vi "StandardStateMachine clock2.vi"() -> ()   [LabVIEW 2014]
doc: "Use this template to build a standard state machine design pattern. Each state executes code and determines which state to transition to. Contrast this design pattern with the User Interface Event Handler pattern, in which code executes in response to user actions. Contrast this design pattern also with the Queued Message Handler pattern, in which each message handling code can queue zero or more new messages.\nNote: This template does not contain the most recent programming guidelines recommended by National Instruments. For a complete, project-based implementation of the Standard State Machine pattern, use the Create Project dialog box instead of this template."
uses:
  second v2.ctl
  minute v2.ctl
  hour v2.ctl
  StateMachineStates clock2.ctl
panel:
  in  "Stop After":i32 format="%.0f Hours"
  in  "Start":bool
  out "minute hand":T1 scale=1.0..59.0
  out "second hand":T2 scale=1.0..59.0
  out "hour hand":T3 scale=0.0..12.0
  out "x+1":i32
  out "HOUR":string
  out "MINUTE":string
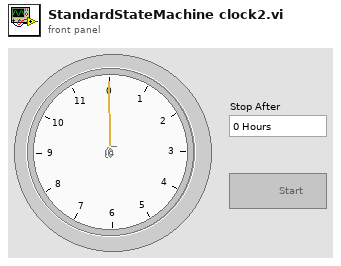
[diagram p1: front panel]
types:
  T1 = typedef "minute v2.ctl" = dbl
  T2 = typedef "second v2.ctl" = dbl
  T3 = typedef "hour v2.ctl" = dbl
  T4 = typedef "StateMachineStates clock2.ctl" = enum16{"Initialize", "normal count", "counting", "Stop"}
  T5 = enum8{"Enabled", "Disabled", "Disabled and Grayed Out"}
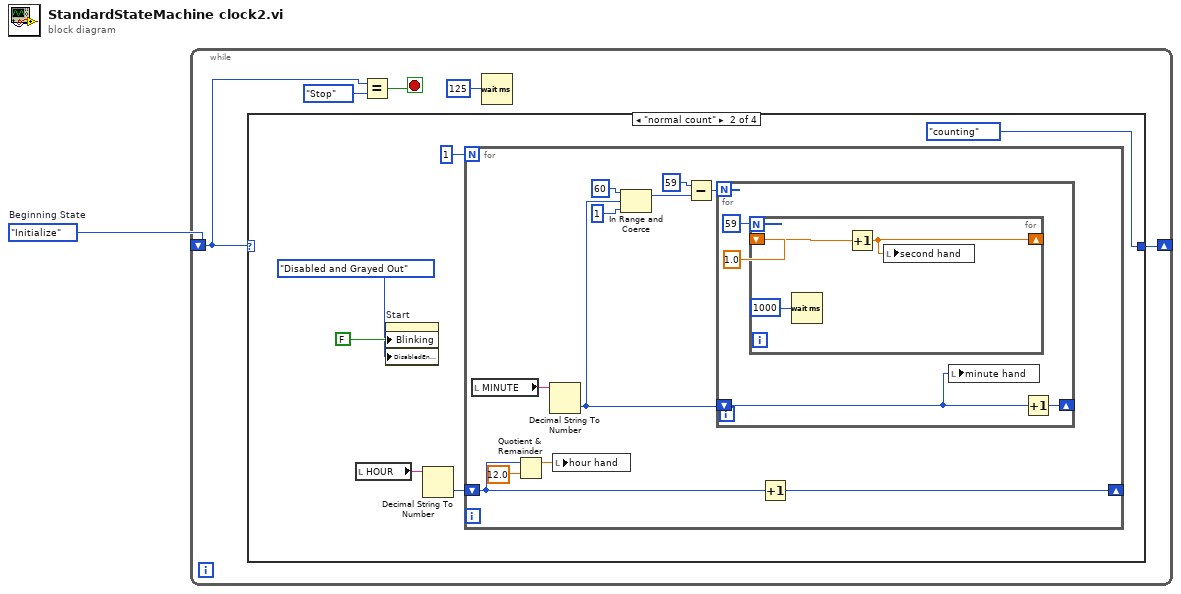
[diagram p0: block diagram]
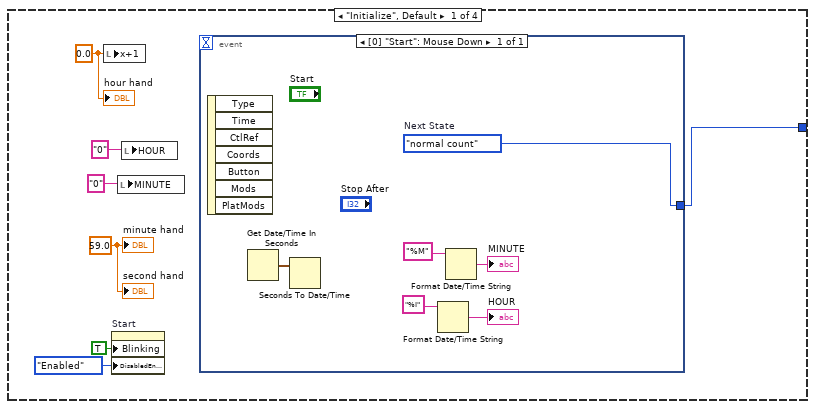
[diagram p2: hidden frame]
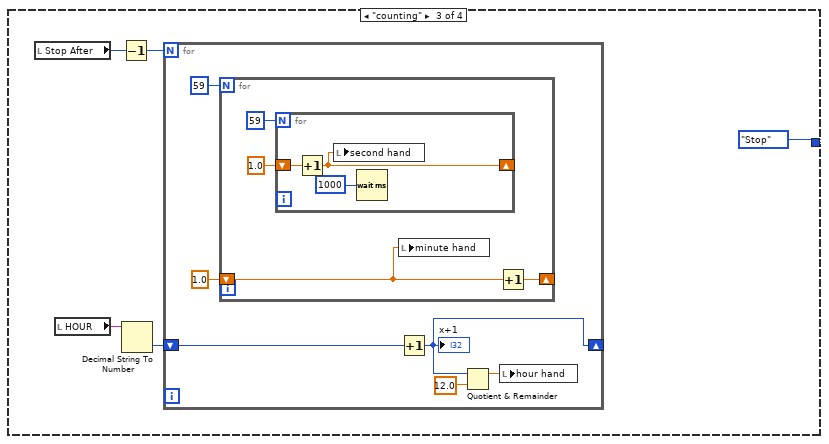
[diagram p3: hidden frame]
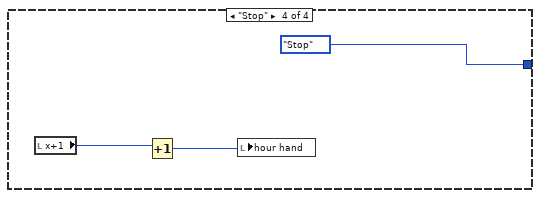
[diagram p4: hidden frame]
diagram:
  w1 = StateMachineStates_clock2."Initialize"  # Beginning State
  n1 = while {
    shift-right: [w3] -> _
    shift-left: w1 -> [w4]
    stop <- w6 stop-if-true
    n2 = case shown="\"normal count\"" w4 {
      tunnel: [w13 StateMachineStates_clock2."counting" ("Next State") StateMachineStates_clock2."Stop" ("Next State") StateMachineStates_clock2."Stop" ("Next State")] -> w3
      frame "Initialize", Default {
        w8 = T3 0.0 ("hour hand")
        w12 = T2 59.0 ("Gauge")
        n3 = local write "x+1"(w8) -> ()
        n4 = property on="Start" class="Bool (strict)"("Blinking"=TRUE ("Visible"), "DisabledEnum"=T5."Enabled" ("Disabled")) -> ()  [unwired: 2 in, 2 out]
        n5 = local write "MINUTE"("0" ("MINUTE")) -> ()
        n6 = local write "HOUR"("0" ("HOUR")) -> ()
        n7 = event shown="[0] \"Start\": Mouse Down" {
          selector: _ -> [_]
          dyn-events: _ -> [_]
          timeout: _ -> [_]
          tunnel: [w19] -> w13
          event "Start": Mouse Down {
            w19 = StateMachineStates_clock2."normal count"  # Next State
            n8 = event-data() -> ()  [unwired: 1 in, 7 out]
            n9 = Get Date/Time In Seconds() -> (seconds since 1Jan1904=w18:timestamp)
            n10 = Seconds To Date/Time(time stamp (now)=w18) -> ()  [unwired: 1 in, 1 out]
            n11 = Format Date/Time String(time format string (%c)="%I") -> (date/time string=→"HOUR":string)  [unwired: 2 in]
            n12 = Format Date/Time String(time format string (%c)="%M") -> (date/time string=→"MINUTE":string)  [unwired: 2 in]
          }
        }
        "second hand" <- w12
        "minute hand" <- w12
        "hour hand" <- w8
      }
      frame "normal count" {
        n13 = local read "HOUR"() -> (w24:string)
        n14 = property on="Start" class="Bool (strict)"("Blinking"=FALSE ("Visible"), "DisabledEnum"=T5."Disabled and Grayed Out" ("Disabled")) -> ()  [unwired: 2 in, 2 out]
        n15 = Decimal String To Number(string=w24) -> (number=w23:i32)  [unwired: 2 in, 1 out]
        n16 = for {
          N: 1 -> [_]
          shift-right: [w32] -> _
          shift-left: w23 -> [w33]
          n17 = local read "MINUTE"() -> (w34:string)
          n18 = Quotient & Remainder(x=w33, y=12.0) -> (x-y*floor(x/y)=w35:dbl)  [unwired: 1 out]
          n19 = Decimal String To Number(string=w34) -> (number=w31:i32)  [unwired: 2 in, 1 out]
          n20 = local write "hour hand"(w35) -> ()
          n21 = In Range and Coerce(upper limit=60, x=w31, lower limit=1) -> (coerced(x)=w27:i32)  [unwired: 1 out]
          n22 = Subtract(x=59 ("y"), y=w27) -> (x-y=w28:i32)
          n23 = for {
            N: w28 -> [_]
            shift-right: [w39] -> _
            shift-left: w31 -> [w40]
            n24 = for {
              N: 59 -> [_]
              shift-right: [w42] -> _
              shift-left: 1.0 -> [w43]
              n25 = Wait (ms)(milliseconds to wait=u32 1000) -> ()  [unwired: 1 out]
              n26 = Increment(x=w43) -> (x+1=w42:dbl)
              n27 = local write "second hand"(w42) -> ()
            }
            n28 = local write "minute hand"(w40) -> ()
            n29 = Increment(x=w40) -> (x+1=w39:i32)
          }
          n30 = Increment(x=w33) -> (x+1=w32:i32)
        }
      }
      frame "counting" {
        n31 = local read "Stop After"() -> (w46:i32)
        n32 = local read "HOUR"() -> (w47:string)
        n33 = Decrement(x=w46) -> (x-1=w45:i32)
        n34 = Decimal String To Number(string=w47) -> (number=w44:i32)  [unwired: 2 in, 1 out]
        n35 = for {
          N: w45 -> [_]
          shift-right: [w49] -> _
          shift-left: w44 -> [w52]
          n36 = for {
            N: 59 -> [_]
            shift-right: [w57] -> _
            shift-left: 1.0 -> [w58]
            n37 = for {
              N: 59 -> [_]
              shift-right: [w60] -> _
              shift-left: 1.0 -> [w61]
              n38 = Increment(x=w61) -> (x+1=w60:dbl)
              n39 = local write "second hand"(w60) -> ()
              n40 = Wait (ms)(milliseconds to wait=u32 1000) -> ()  [unwired: 1 out]
            }
            n41 = local write "minute hand"(w58) -> ()
            n42 = Increment(x=w58) -> (x+1=w57:dbl)
          }
          n43 = Increment(x=w52) -> (x+1=w49:i32)
          "x+1" <- w49
          n44 = Quotient & Remainder(x=w49, y=12.0) -> (x-y*floor(x/y)=w53:dbl)  [unwired: 1 out]
          n45 = local write "hour hand"(w53) -> ()
        }
      }
      frame "Stop" {
        n46 = local read "x+1"() -> (w62:i32)
        n47 = Increment(x=w62) -> (x+1=w63:i32)
        n48 = local write "hour hand"(w63) -> ()
      }
    }
    n49 = Equal?(x=w4, y=StateMachineStates_clock2."Stop" ("States")) -> (x = y?=w6:bool)
    n50 = Wait (ms)(milliseconds to wait=u32 125) -> ()  [unwired: 1 out]
  }
